vi "Go_to_Init.vi"(8 "error in (no error)":errorcluster, 11 "Demo_States in":refnum<class "Demo_States.lvclass">) -> (0 "error out":errorcluster, 3 "State out":refnum<class "State Actor.lvclass">)   [LabVIEW 2025, in "Demo_States.lvlib" / "Demo_States.lvclass"]
uses:
  Demo_States.lvclass
  Demo_States.lvclass/Demo_States.ctl
  C:/Program Files (x86)/National Instruments/LabVIEW 2025/vi.lib/ni/Actors/State Actor/State Actor/State Actor.lvclass
  C:/Program Files (x86)/National Instruments/LabVIEW 2025/vi.lib/ActorFramework/Actor/Actor.lvclass
  C:/Users/halstead_rideriver/Documents/Labview_Practice/ATM_Machine_Actor Framework/ATM_ACTORFW/Demo_States/Demo_States/Demo_States.lvclass
  Init_cls/Init_cls.lvclass
  C:/Users/halstead_rideriver/Documents/Labview_Practice/ATM_Machine_Actor Framework/ATM_ACTORFW/Demo_States/Init_cls/Init_cls.lvclass
  <vilib>/ni/Actors/State Actor/State Actor/State Actor.lvclass
  <vilib>/ActorFramework/Actor/Actor.lvclass
  demo Messages/Log State Msg/Log State Msg.lvclass
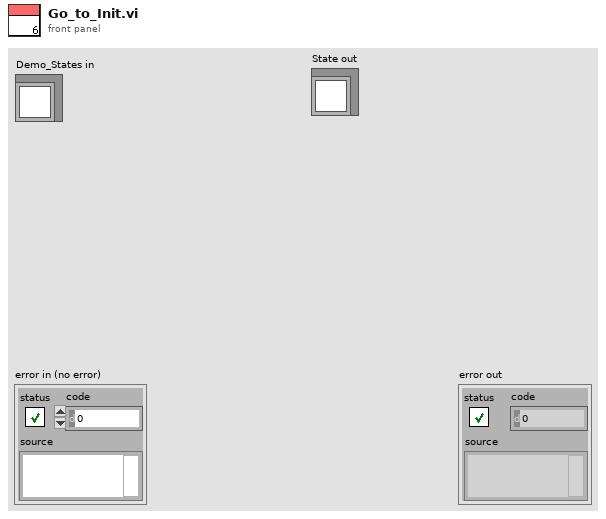
[diagram p1: front panel]
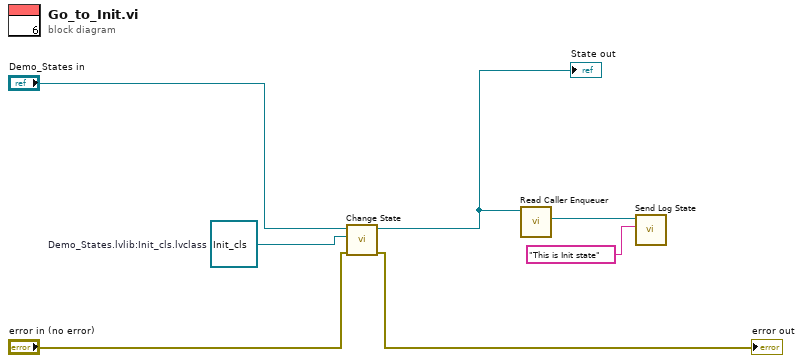
[diagram p0: block diagram]
diagram:
  w4 = refnum<class "Init_cls.lvclass"> refnum  # Demo_States.lvlib:Init_cls.lvclass
  n1 = call <vilib>:"Change State.vi"("error in (no error)"="error in (no error)", "New State in"=w4, "State in"="Demo_States in") -> ("error out"=→"error out":errorcluster, "State out"=w3:refnum<class "State Actor.lvclass">)  [unwired: 7 in]
  "State out" <- w3
  n2 = call <vilib>:"Read Caller Enqueuer.vi"("Actor"=w3) -> ("Caller Enqueuer"=w2:refnum<class "Message Enqueuer.lvclass">)  [unwired: 10 in]
  n3 = call "Send Log State.vi"("State"="This is Init state", "Message Enqueuer"=w2) -> ()  [unwired: 8 in, 2 out]
